vi "GEECS scan path to local scan path.vi"(8 "error in (no error)":errorcluster, 10 "LocalSavePath":path=path "C:/data", 11 "Path":path) -> (0 "error out":errorcluster, 3 "local path for scans":path)   [LabVIEW 2020]
panel:
  out "stripped path":path
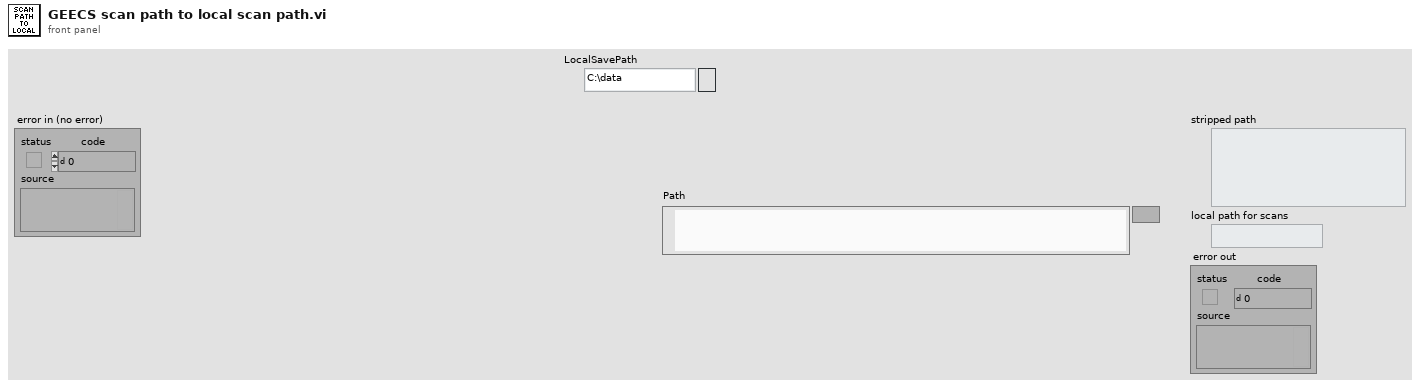
[diagram p1: front panel]
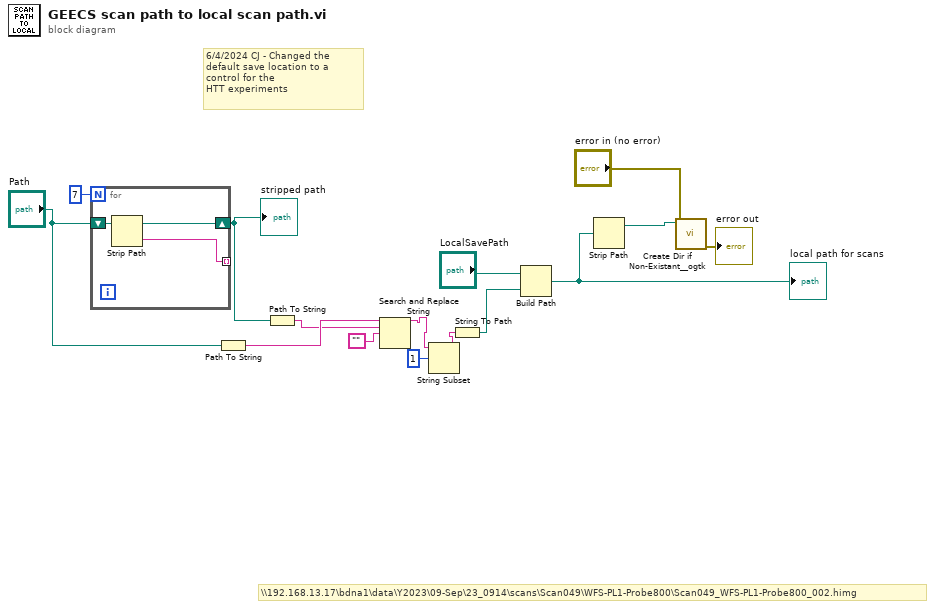
[diagram p0: block diagram]
diagram:
  # "6/4/2024 CJ - Changed the default save location to a control for the \nHTT experiments"
  # "\\\\192.168.13.17\\bdna1\\data\\Y2023\\09-Sep\\23_0914\\scans\\Scan049\\WFS-PL1-Probe800\\Scan049_WFS-PL1-Probe800_002.himg"
  n1 = for {
    N: 7 -> [_]
    shift-right: [w17] -> w13
    shift-left: "Path" -> [w18]
    tunnel: [w16] -> _ mode=indexing
    n2 = Strip Path(path=w18) -> (stripped path=w17:path, name=w16:string)
  }
  "stripped path" <- w13
  n3 = Path To String(path="Path") -> (string=w12:string)
  n4 = Path To String(path=w13) -> (string=w11:string)
  n5 = Search and Replace String(input string=w12, search string=w11, replace string="") -> (result string=w8:string)  [unwired: 5 in, 3 out]
  n6 = String Subset(string=w8, offset (0)=1) -> (substring=w6:string)  [unwired: 1 in]
  n7 = String To Path(string=w6) -> (path=w9:path)
  n8 = Build Path(base path="LocalSavePath", name or relative path=w9) -> (appended path=w5:path)
  "local path for scans" <- w5
  n9 = Strip Path(path=w5) -> (stripped path=w4:path)  [unwired: 1 out]
  n10 = call "Create Dir if Non-Existant__ogtk.vi"("error in (no error)"="error in (no error)", "Directory Path"=w4) -> ("error out"=→"error out":errorcluster)  [unwired: 7 in, 2 out]
